vi "Teleop-MAY.vi"(10 "Match Info":T2={"Autonomous Elapsed Seconds"=0.0, "TeleOp Elapsed Seconds"=0.0, "Disabled Elapsed Seconds"=0.0, "Visited Autonomous"=FALSE, "Visited TeleOp"=FALSE, "Visited Disabled"=FALSE, "Autonomous Settings"={"Autonomous Style"=enum."Independent", "VI Refnum"=refnum}}, 11 "Call Context":T3) -> ()   [LabVIEW 2017]
doc: "This VI is called for each TeleOp packet received from the DS where the robot is not disabled. It is often used to read from the joysticks and update I/O or to update setpoints for timed control loops. It should complete and return within 20 milliseconds or it may miss DS packets."
uses:
  <vilib>/Rock Robotics/WPI/DriverStation/WPI_DriverStationDerivedRobotMode.ctl
  <vilib>/Rock Robotics/WPI/DriverStation/WPI_DriverStationMatch Info.ctl
  Systems/Shooter/ENUM_CMD Select.ctl
  TypeDefs/ENUM_Overloard States.ctl
  Systems/Shooter/Cluster_CMD to SM Data.ctl
  TypeDefs/ENUM_Overloard Shooter States.ctl
  Systems/Controller/Global_Data Out.vi
  Systems/Shooter/Global_CMD to SM Data.vi
  Systems/Controller/Controller.lvlib
  Systems/Shooter/Shooter.lvlib
panel:
  in  "Wheel RPM":dbl
  in  "Hood Position":dbl
  in  "Select":T1=enum."Encoder Both"
  in  "Hood VBus":dbl
  in  "Wheel VBus":dbl min=-1.0 max=1.0 step=0.01
  in  "Hopper Empty?":bool
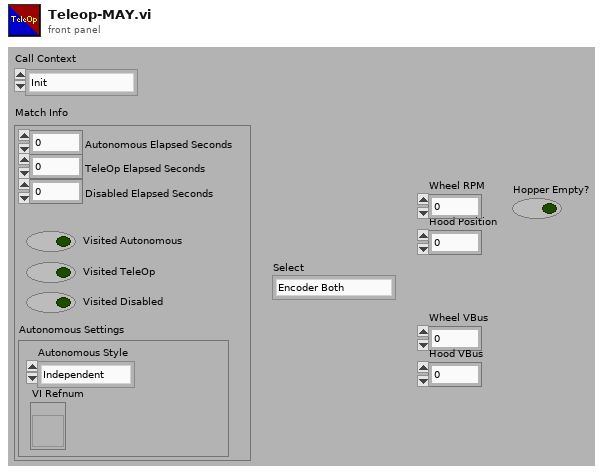
[diagram p1: front panel]
types:
  T1 = typedef "Shooter.lvlib/ENUM_CMD Select.ctl" = enum16{"Stop", "Manual VBus", "Encoder Hood Only", "Encoder Wheel Only", "Encoder Both"}
  T2 = typedef "WPI_DriverStationMatch Info.ctl" = cluster{"Autonomous Elapsed Seconds":dbl, "TeleOp Elapsed Seconds":dbl, "Disabled Elapsed Seconds":dbl, "Visited Autonomous":bool, "Visited TeleOp":bool, "Visited Disabled":bool, "Autonomous Settings":cluster{"Autonomous Style":enum16{"Iterative", "Independent"}, "VI Refnum":refnum<vi>}}
  T3 = typedef "WPI_DriverStationDerivedRobotMode.ctl" = enum16{"Init", "Execute", "Stop"}
  T4 = typedef "ENUM_Overloard States.ctl" = enum16{"Idle", "Manual", "High Shot", "Low Shot", "Place Gear", "Climb"}
  T5 = typedef "Shooter.lvlib/Cluster_CMD to SM Data.ctl" = cluster{"Select":T1, "Wheel VBus":dbl, "Wheel RPM":dbl, "Hood VBus":dbl, "Hood Position":dbl}
  T6 = typedef "ENUM_Overloard Shooter States.ctl" = enum16{"Idle", "Locate Target", "Wait To Be in Position", "Shooting", "Complete"}
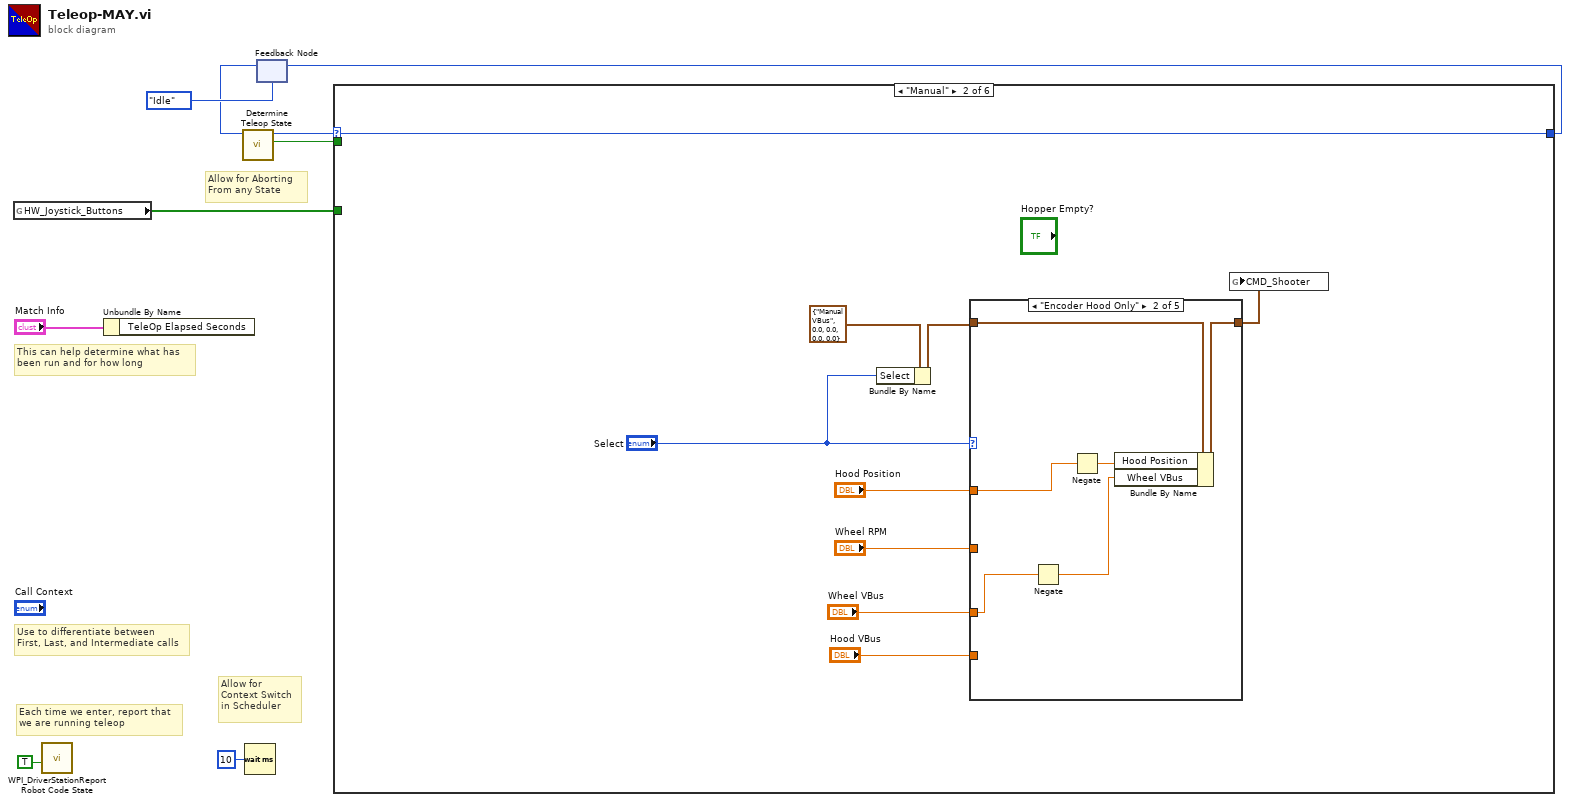
[diagram p0: block diagram]
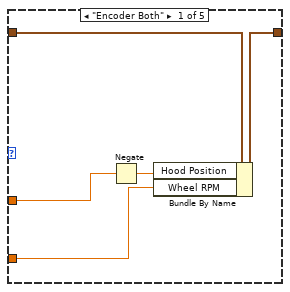
[diagram p3: hidden frame]
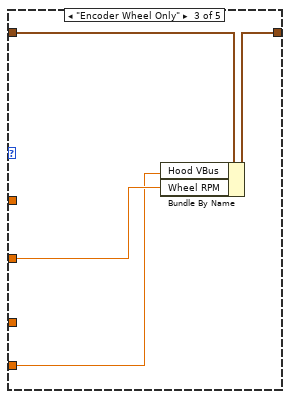
[diagram p4: hidden frame]
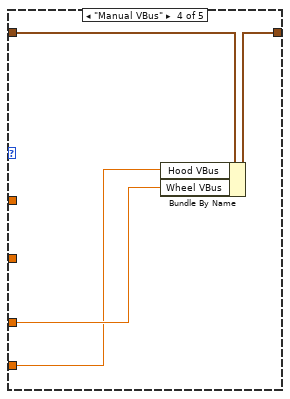
[diagram p5: hidden frame]
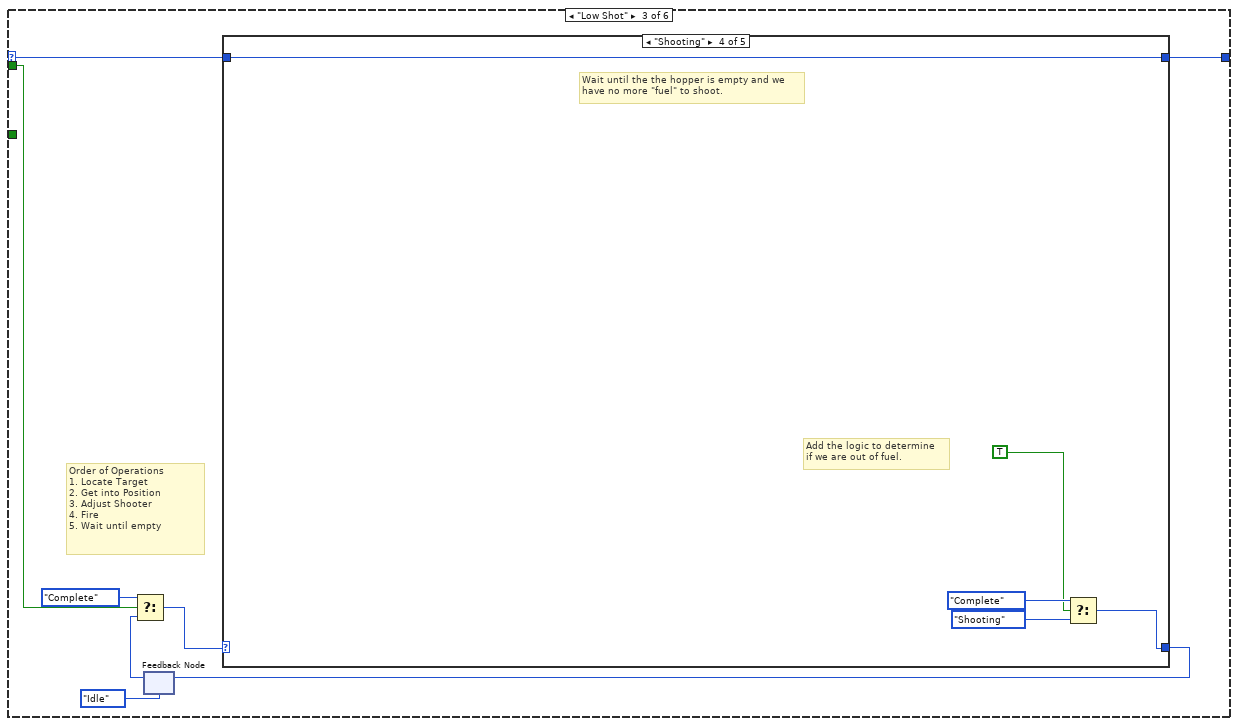
[diagram p7: hidden frame]
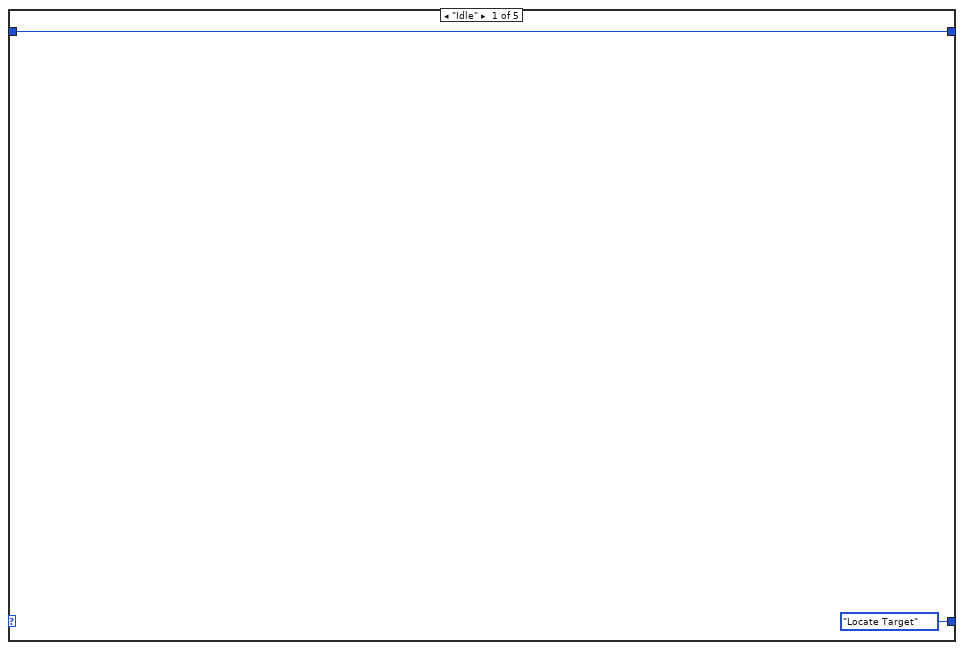
[diagram p8: hidden frame]
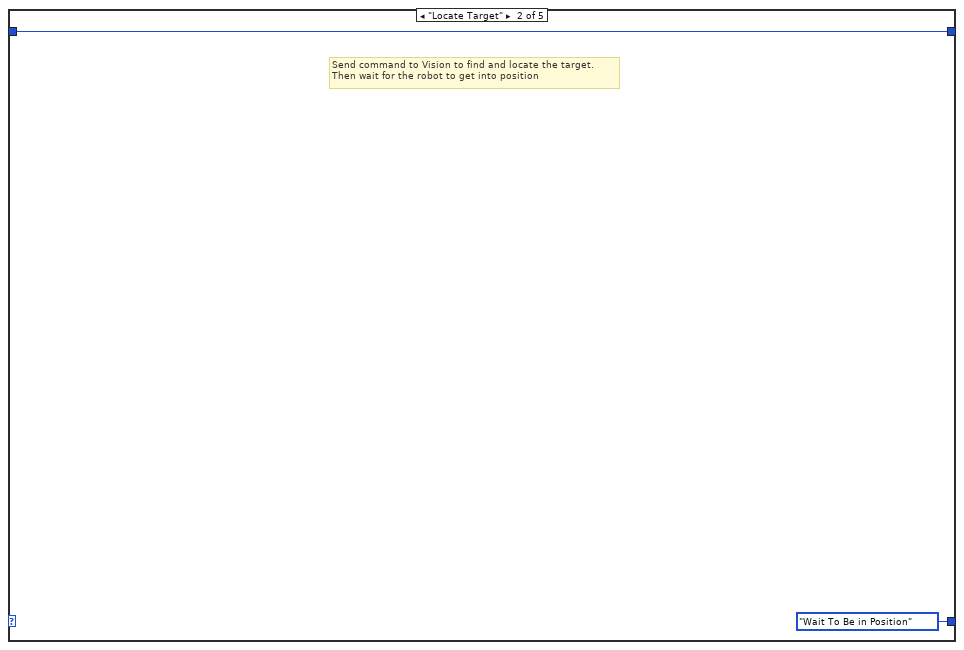
[diagram p9: hidden frame]
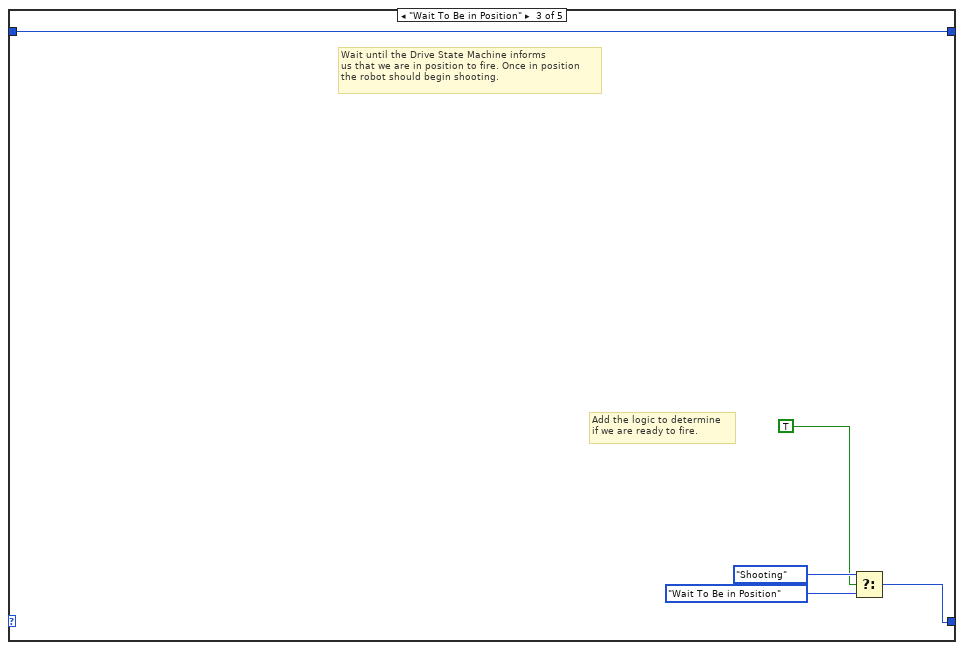
[diagram p10: hidden frame]
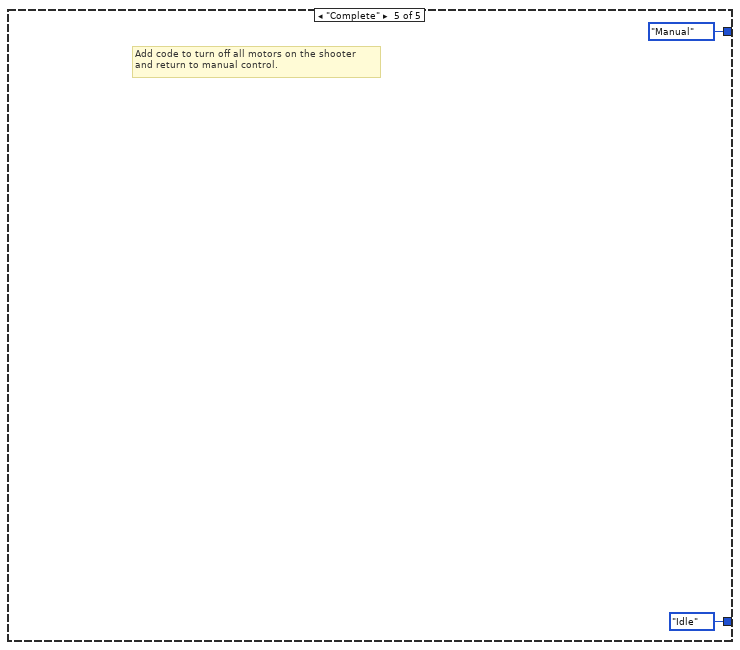
[diagram p11: hidden frame]
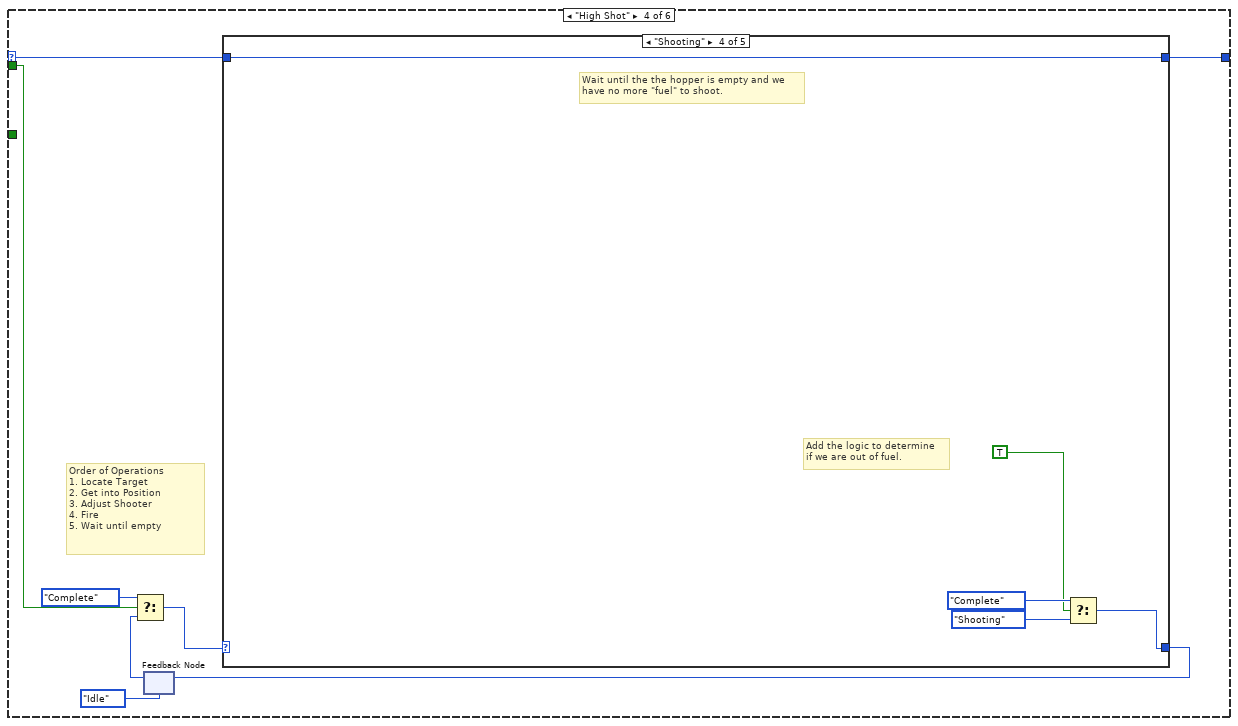
[diagram p12: hidden frame]
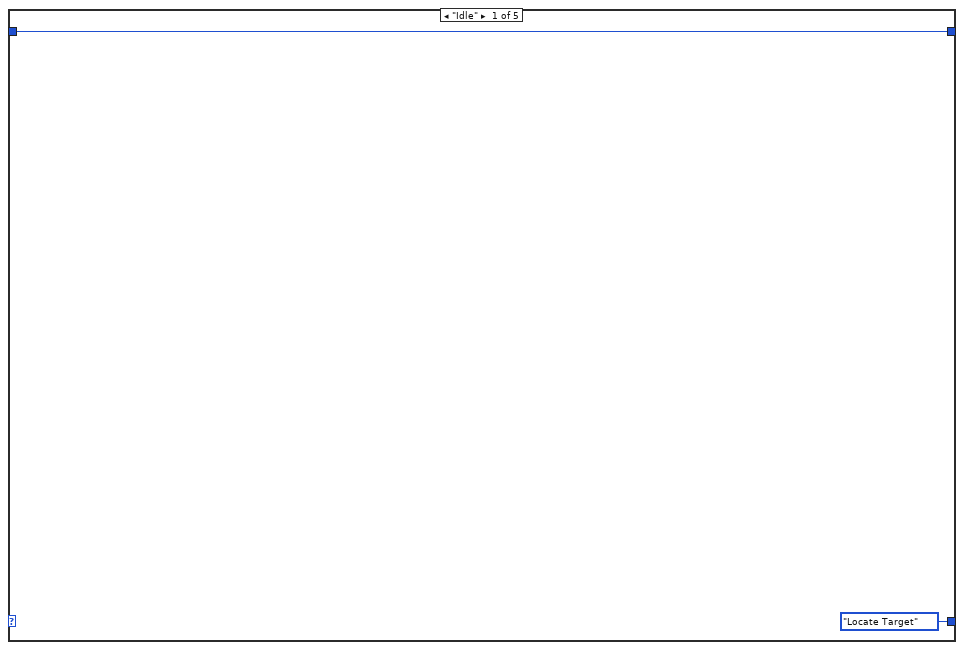
[diagram p13: hidden frame]
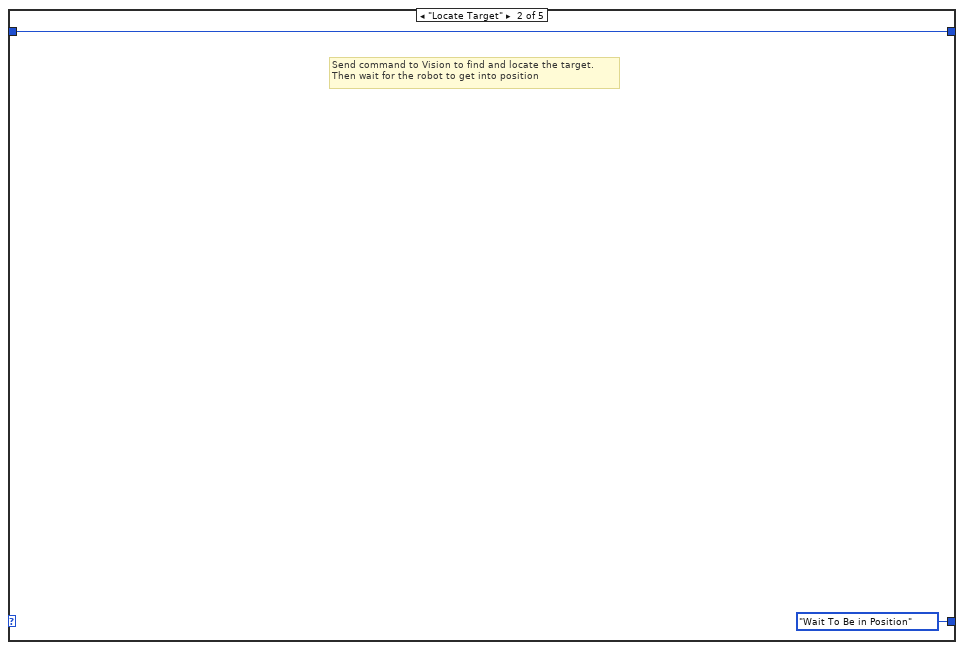
[diagram p14: hidden frame]
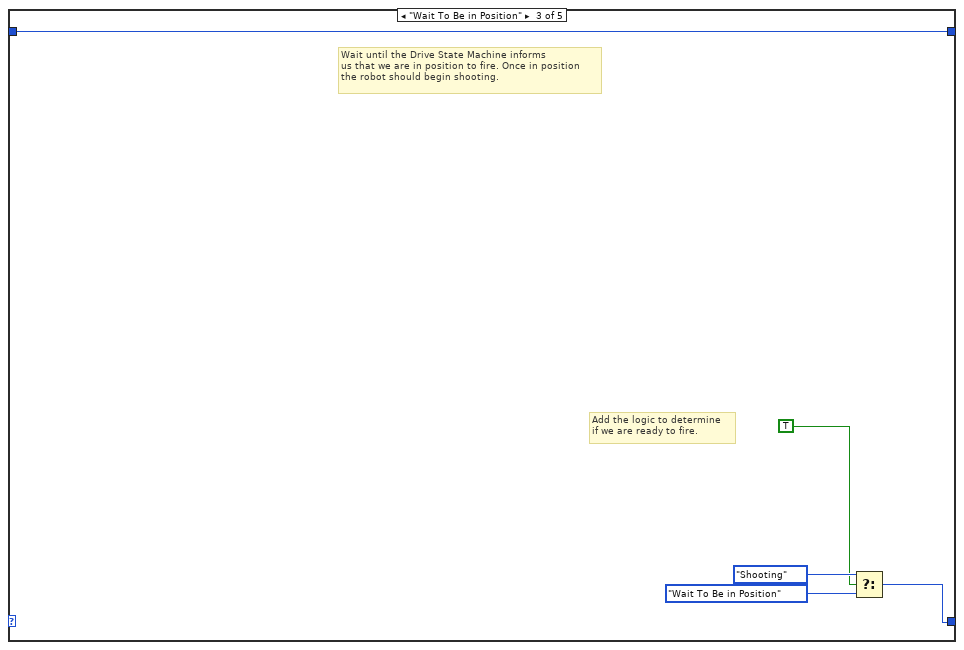
[diagram p15: hidden frame]
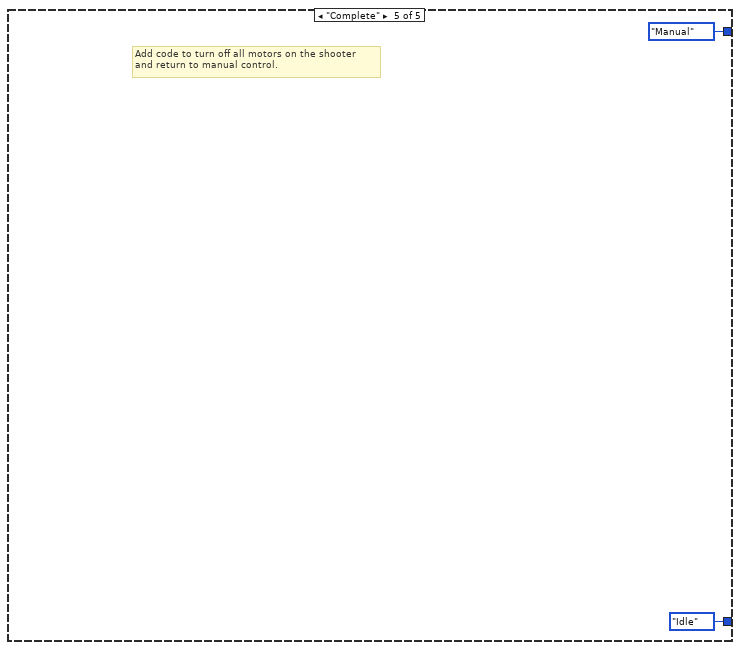
[diagram p16: hidden frame]
diagram:
  # "Allow for Aborting\nFrom any State"
  # "Allow for\nContext Switch\nin Scheduler"
  # "Each time we enter, report that\nwe are running teleop"
  # "Use to differentiate between\nFirst, Last, and Intermediate calls"
  # "This can help determine what has\nbeen run and for how long"
  n1 = global read "Global_Data Out.vi" "HW_Joystick_Buttons"() -> (w5:bool[])
  n2 = call <vilib>:"WPI_DriverStationReport Robot Code State.vi"("TeleOp"=TRUE ("Autonomous")) -> ()  [unwired: 10 in, 1 out]
  n3 = Unbundle By Name("Match Info") -> ()  [unwired: 1 out]
  n4 = Wait (ms)(milliseconds to wait=u32 10) -> ()  [unwired: 1 out]
  n5 = feedback #1(ENUM_Overloard_States."Idle" ("Teleop State")) -> (w3:T4)
  n6 = call "Determine Teleop State.vi"("Teleop State"=w3) -> ("Abort"=w1:bool, "Teleop State"=w2:T4)  [unwired: 9 in]
  n7 = case shown="\"Manual\"" w2 {
    selector: w2 -> [w10 w19 w45 w69 w88 w89]
    tunnel: [w10 w19 w44 w68 w88 w89] -> w7
    tunnel: w5 -> [_ _ _ _ _ _]
    tunnel: w1 -> [_ _ w43 w67 _ _]
    frame "Idle" {
      # "Do nothing"
    }
    frame "Manual" {
      n8 = Bundle By Name(cluster=T5 {"Select"=enum."Manual VBus", "Wheel VBus"=0.0, "Wheel RPM"=0.0, "Hood VBus"=0.0, "Hood Position"=0.0} ("CMD_Shooter"), "Select"="Select") -> (w16:T5)
      n9 = case shown="\"Encoder Hood Only\"" "Select" {
        tunnel: w16 -> [w24 w30 w34 w38 w39]
        tunnel: [w23 w29 w33 w37 w39] -> w18
        tunnel: "Hood Position" -> [w21 w27 _ _ _]
        tunnel: "Wheel RPM" -> [w20 _ w32 _ _]
        tunnel: "Wheel VBus" -> [_ w26 _ w36 _]
        tunnel: "Hood VBus" -> [_ _ w31 w35 _]
        frame "Encoder Both" {
          n10 = Negate(x=w21) -> (-x=w22:dbl)
          n11 = Bundle By Name(cluster=w24, "Hood Position"=w22, "Wheel RPM"=w20) -> (w23:T5)
        }
        frame "Encoder Hood Only" {
          n12 = Negate(x=w26) -> (-x=w25:dbl)
          n13 = Negate(x=w27) -> (-x=w28:dbl)
          n14 = Bundle By Name(cluster=w30, "Hood Position"=w28, "Wheel VBus"=w25) -> (w29:T5)
        }
        frame "Encoder Wheel Only" {
          n15 = Bundle By Name(cluster=w34, "Hood VBus"=w31, "Wheel RPM"=w32) -> (w33:T5)
        }
        frame "Manual VBus" {
          n16 = Bundle By Name(cluster=w38, "Hood VBus"=w35, "Wheel VBus"=w36) -> (w37:T5)
        }
        frame "Stop" {
        }
      }
      n17 = global write "Global_CMD to SM Data.vi" "CMD_Shooter"(w18) -> ()
    }
    frame "Low Shot" {
      # "Order of Operations\n1. Locate Target\n2. Get into Position\n3. Adjust Shooter\n4. Fire\n5. Wait until empty"
      n18 = feedback #2(ENUM_Overloard_Shooter_States."Idle" ("Shooter States")) -> (w42:T6)
      n19 = Select(t=ENUM_Overloard_Shooter_States."Complete" ("Shooter States"), s=w43, f=w42) -> (s? t:f=w41:T6)
      n20 = case shown="\"Shooting\"" w41 {
        tunnel: [ENUM_Overloard_Shooter_States."Locate Target" ("Shooter States") ENUM_Overloard_Shooter_States."Wait To Be in Position" ("Shooter States") w55 w60 ENUM_Overloard_Shooter_States."Idle" ("Shooter States")] -> w47
        tunnel: w45 -> [w49 w51 w56 w61 _]
        tunnel: [w49 w51 w56 w61 ENUM_Overloard_States."Manual" ("Teleop State")] -> w44
        frame "Idle" {
        }
        frame "Locate Target" {
          # "Send command to Vision to find and locate the target.\nThen wait for the robot to get into position"
        }
        frame "Wait To Be in Position" {
          # "Add the logic to determine\nif we are ready to fire."
          # "Wait until the Drive State Machine informs\nus that we are in position to fire. Once in position\nthe robot should begin shooting."
          n21 = Select(t=ENUM_Overloard_Shooter_States."Shooting" ("Shooter States"), s=TRUE, f=ENUM_Overloard_Shooter_States."Wait To Be in Position" ("Shooter States")) -> (s? t:f=w55:T6)
        }
        frame "Shooting" {
          # "Add the logic to determine\nif we are out of fuel."
          # "Wait until the the hopper is empty and we\nhave no more \"fuel\" to shoot."
          n22 = Select(t=ENUM_Overloard_Shooter_States."Complete" ("Shooter States"), s=TRUE, f=ENUM_Overloard_Shooter_States."Shooting" ("Shooter States")) -> (s? t:f=w60:T6)
        }
        frame "Complete" {
          # "Add code to turn off all motors on the shooter\nand return to manual control."
        }
      }
      n23 = feedback-in #2(w47) -> ()
    }
    frame "High Shot" {
      # "Order of Operations\n1. Locate Target\n2. Get into Position\n3. Adjust Shooter\n4. Fire\n5. Wait until empty"
      n24 = feedback #3(ENUM_Overloard_Shooter_States."Idle" ("Shooter States")) -> (w66:T6)
      n25 = Select(t=ENUM_Overloard_Shooter_States."Complete" ("Shooter States"), s=w67, f=w66) -> (s? t:f=w65:T6)
      n26 = case shown="\"Shooting\"" w65 {
        tunnel: [ENUM_Overloard_Shooter_States."Locate Target" ("Shooter States") ENUM_Overloard_Shooter_States."Wait To Be in Position" ("Shooter States") w79 w84 ENUM_Overloard_Shooter_States."Idle" ("Shooter States")] -> w71
        tunnel: w69 -> [w73 w75 w80 w85 _]
        tunnel: [w73 w75 w80 w85 ENUM_Overloard_States."Manual" ("Teleop State")] -> w68
        frame "Idle" {
        }
        frame "Locate Target" {
          # "Send command to Vision to find and locate the target.\nThen wait for the robot to get into position"
        }
        frame "Wait To Be in Position" {
          # "Add the logic to determine\nif we are ready to fire."
          # "Wait until the Drive State Machine informs\nus that we are in position to fire. Once in position\nthe robot should begin shooting."
          n27 = Select(t=ENUM_Overloard_Shooter_States."Shooting" ("Shooter States"), s=TRUE, f=ENUM_Overloard_Shooter_States."Wait To Be in Position" ("Shooter States")) -> (s? t:f=w79:T6)
        }
        frame "Shooting" {
          # "Add the logic to determine\nif we are out of fuel."
          # "Wait until the the hopper is empty and we\nhave no more \"fuel\" to shoot."
          n28 = Select(t=ENUM_Overloard_Shooter_States."Complete" ("Shooter States"), s=TRUE, f=ENUM_Overloard_Shooter_States."Shooting" ("Shooter States")) -> (s? t:f=w84:T6)
        }
        frame "Complete" {
          # "Add code to turn off all motors on the shooter\nand return to manual control."
        }
      }
      n29 = feedback-in #3(w71) -> ()
    }
    frame "Place Gear" {
      # "See the High and Low shot for the\nway to implement the state machine."
      # "Order of Operations\n1. Find Target\n2: Get into position\n3. Place Peg\n4: Drop gear on peg\n5. Backup"
    }
    frame "Climb" {
      # "See the High and Low shot for the\nway to implement the state machine."
    }
  }
  n30 = feedback-in #1(w7) -> ()
